vi "Read Attributes.vi"(11 "VI Information Changed Msg":refnum<class "VI Information Changed Msg.lvclass">) -> (2 "Payload":cluster{"VI Infomation":T1})   [LabVIEW 2015, in "Interface.lvlib" / "VI Information Changed Msg.lvclass"]
uses:
  VI Information Changed Msg.lvclass
  Interface/Controls/VI Infomation.ctl
  Interface/Interface.lvlib
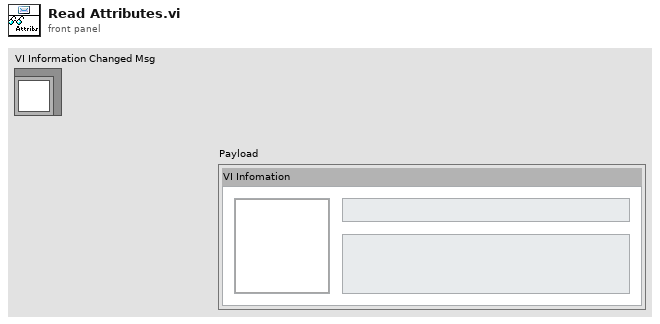
[diagram p1: front panel]
types:
  T1 = typedef "Interface.lvlib/VI Infomation.ctl" = cluster{"VI Name":string, "VI Description":string, "VI Icon":picture}
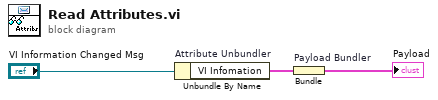
[diagram p0: block diagram]
diagram:
  n1 = Unbundle By Name "Attribute Unbundler"("VI Information Changed Msg") -> ("VI Infomation"=w1:T1)
  n2 = Bundle "Payload Bundler"("VI Infomation"=w1) -> (→"Payload":cluster{"VI Infomation":T1})  [unwired: 1 in]
